vi "Subscribe SensorView.vi"(8 "error in (no error)":errorcluster, 9 "HostType":T1, 10 "SensorView Enqueuer":refnum<class "Message Enqueuer.lvclass">, 11 "Sensor in":refnum<class "Sensor.lvclass">) -> (0 "error out":errorcluster, 3 "Sensor out":refnum<class "Sensor.lvclass">)   [LabVIEW 2012, in "Sensor Definition.lvlib" / "Sensor.lvclass"]
uses:
  Sensor.lvclass
  <vilib>/ActorFramework/Message Enqueuer/Message Enqueuer.lvclass
  HostType.ctl
  Sensor.lvclass/Sensor.ctl
  SensorView Messages/Update Sensor Info Msg/Update Sensor Info Msg.lvclass/Update Sensor Info Msg.ctl
  <vilib>/ActorFramework/Message Enqueuer/Message Enqueuer.lvclass/Message Enqueuer.ctl
  Read Listening SensorViews.vi
  Read SensorInfo.vi
  Read Listening HostTypes.vi
  Write Listening SensorViews.vi
  Write Listening HostTypes.vi
  <vilib>/ActorFramework/Message Enqueuer/Enqueue.vi
  <vilib>/ActorFramework/Message Priority Queue/Priority Enqueue.vi
  SensorInfo.lvclass
  SensorView Messages/Update Sensor Info Msg/Update Sensor Info Msg.lvclass
  Sensor Definition.lvlib
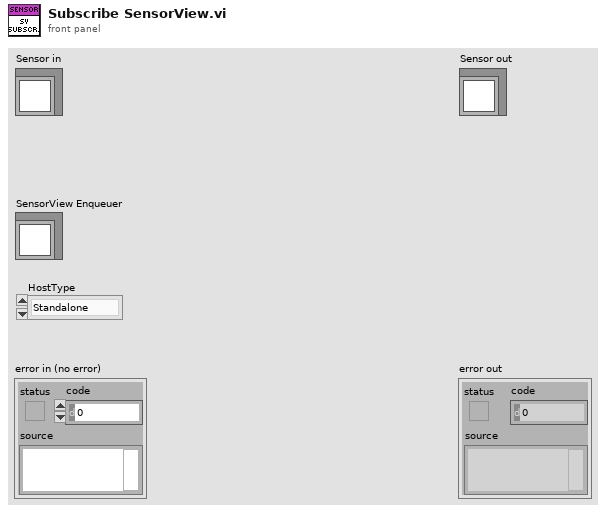
[diagram p1: front panel]
types:
  T1 = typedef "Sensor Definition.lvlib/HostType.ctl" = enum16{"Standalone", "Grid", "MainPane"}
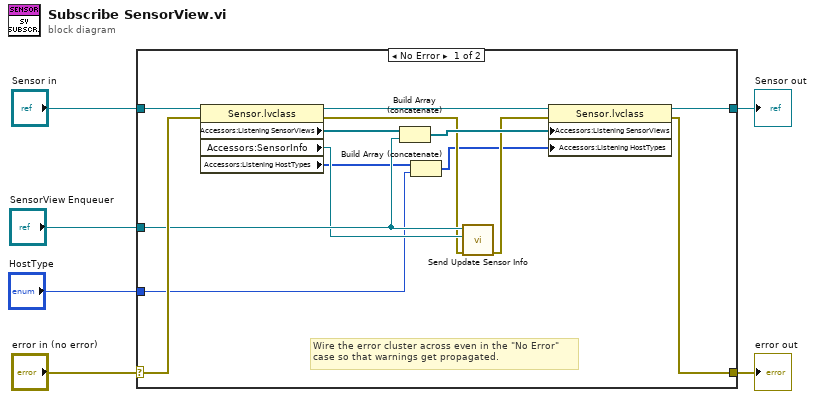
[diagram p0: block diagram]
diagram:
  n1 = case shown="No Error" "error in (no error)" {
    selector: "error in (no error)" -> [w17 w22]
    tunnel: [w16 w22] -> w5
    tunnel: [w19 w21] -> w3
    tunnel: "Sensor in" -> [w20 w21]
    tunnel: "SensorView Enqueuer" -> [w13 _]
    tunnel: "HostType" -> [w7 _]
    frame No Error {
      # "Wire the error cluster across even in the \"No Error\"\ncase so that warnings get propagated."
      n2 = property class="Sensor.lvclass"(reference=w20, error in=w17) -> (reference out=w18:refnum<class "Sensor.lvclass">, error out=w11:errorcluster, "Accessors:Listening SensorViews"=w15:refnum<class "Message Enqueuer.lvclass">[], "Accessors:SensorInfo"=w12:refnum<class "SensorInfo.lvclass">, "Accessors:Listening HostTypes"=w9:T1[])
      n3 = Build Array (concatenate)(w15, w13) -> (w14:refnum<class "Message Enqueuer.lvclass">[])
      n4 = Build Array (concatenate)(w9, w7) -> (w8:T1[])
      n5 = call "Send Update Sensor Info.vi"("error in (no error)"=w11, "SensorInfo"=w12, "Message Enqueuer"=w13) -> ("error out"=w10:errorcluster)  [unwired: 7 in, 1 out]
      n6 = property class="Sensor.lvclass"(reference=w18, error in=w10, "Accessors:Listening SensorViews"=w14, "Accessors:Listening HostTypes"=w8) -> (reference out=w19:refnum<class "Sensor.lvclass">, error out=w16:errorcluster)
    }
    frame Error {
    }
  }
  "error out" <- w5
  "Sensor out" <- w3
